vi "Update_Ch_data_file.vi"(5 "Range":enum16{"All Ch data", "The last few rows"}(ring), 7 "Channel to search on":string, 8 "Start of read offset (chars.: 0)":i32, 9 "New Row values":string[](array[string]), 10 "Present Channels":string[](array[string]), 11 "Filename":path) -> ()   [LabVIEW 2014]
panel:
  out "exists?":bool
  out "Merged?":bool
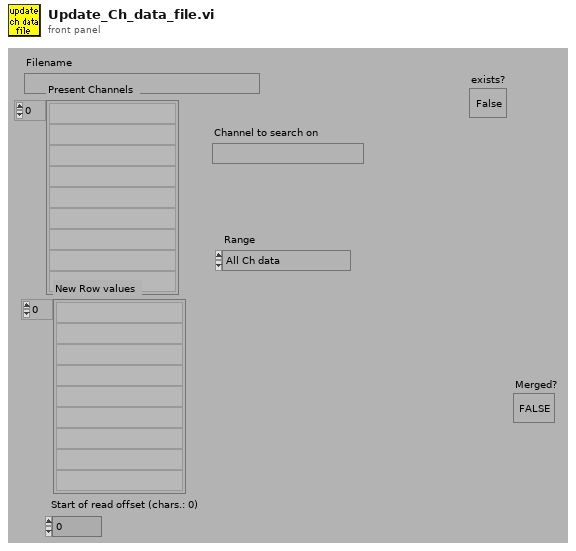
[diagram p1: front panel]
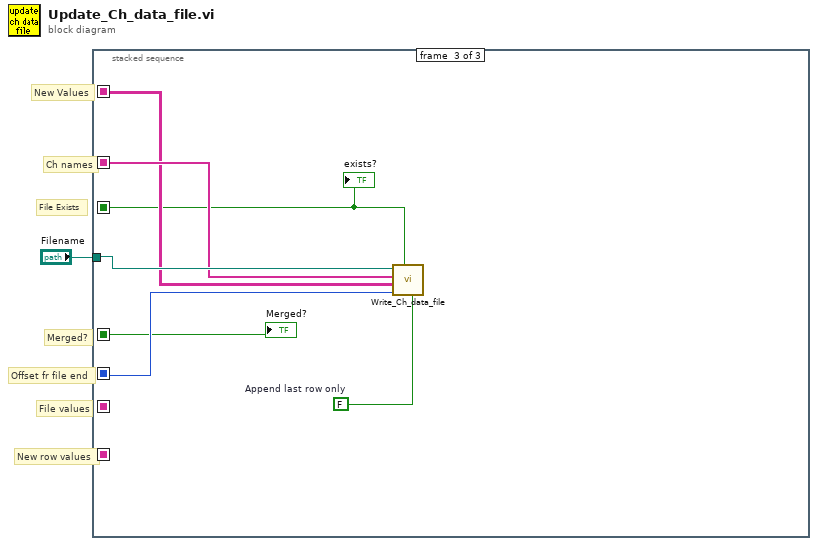
[diagram p0: block diagram]
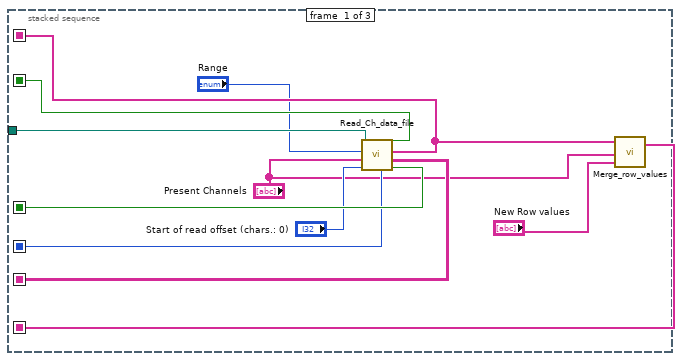
[diagram p2: hidden frame]
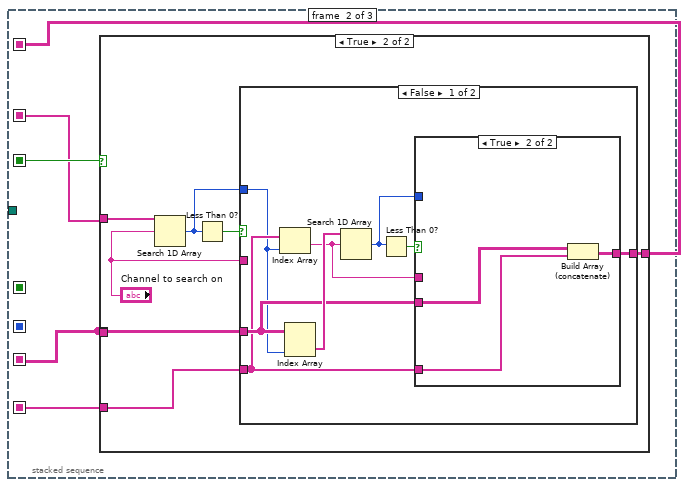
[diagram p3: hidden frame]
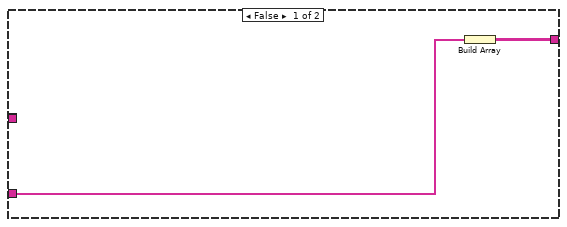
[diagram p4: hidden frame]
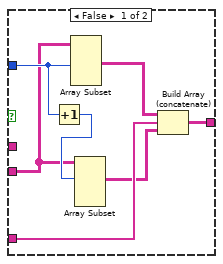
[diagram p5: hidden frame]
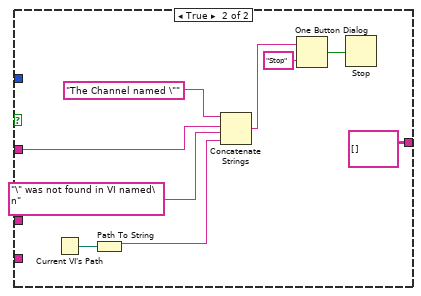
[diagram p6: hidden frame]
diagram:
  # "New row values"
  # "New Values"
  # "File values"
  # "Offset fr file end"
  # "Ch names"
  # "File Exists"
  # "Merged?"
  n1 = stacked-sequence {
    seq-local: [w8 _ _] -> [_ w13 _]
    seq-local: [_ w17 _] -> [_ _ w57]
    seq-local: [w12 _ _] -> [_ _ w54]
    seq-local: [w11 _ _] -> [_ w16 w56]
    seq-local: [w4 _ _] -> [_ w15 w59]
    seq-local: [w9 _ _] -> [_ _ w58]
    seq-local: [w3 _ _] -> [_ w14 _]
    tunnel: "Filename" -> [w10 _ w60]
    frame #0 {
      n2 = call "Read_Ch_data_file.vi"("Start of read offset (chars.: 0)"="Start of read offset (chars.: 0)", "Present Channels"="Present Channels", "Output"="Range", "Filename"=w10) -> ("Merged?"=w12:bool, "Channel Values"=w8:string[][], "Merged Channels"=w4:string[], "exists?"=w11:bool, "Offset from File End"=w9:i32)  [unwired: 1 in]
      n3 = call "Merge_row_values.vi"("Present Row values"="New Row values", "Present Channels"="Present Channels", "Desired Channels"=w4) -> ("Desired Row values"=w3:string[])  [unwired: 1 out]
    }
    frame #1 {
      n4 = case shown="True" w16 {
        tunnel: w15 -> [_ w24]
        tunnel: w13 -> [_ w23]
        tunnel: w14 -> [w18 w22]
        tunnel: [w19 w21] -> w17
        tunnel: w13 -> [_ _]
        frame False {
          n5 = Build Array(w18) -> (w19:string[][])
        }
        frame True {
          n6 = Search 1D Array(1D array=w24, element="Channel to search on") -> (index of element=w25:i32)  [unwired: 1 out]
          n7 = Less Than 0?(x=w25) -> (x < 0?=w26:bool)
          n8 = case shown="False" w26 {
            tunnel: "Channel to search on" -> [_ w46]
            tunnel: w25 -> [w28 _]
            tunnel: w23 -> [w31 _]
            tunnel: w22 -> [w29 _]
            tunnel: [w30 string[][] []] -> w21
            frame False {
              n9 = Index Array(array=w29, index=w28) -> (element=w27:string)
              n10 = Index Array(array=w31, index (col)=w28) -> (element=w34:string[])  [unwired: 1 in]
              n11 = Search 1D Array(1D array=w34, element=w27) -> (index of element=w32:i32)  [unwired: 1 out]
              n12 = Less Than 0?(x=w32) -> (x < 0?=w33:bool)
              n13 = case shown="True" w33 {
                tunnel: w27 -> [_ _]
                tunnel: w32 -> [w39 _]
                tunnel: w31 -> [w37 w43]
                tunnel: w29 -> [w40 w42]
                tunnel: [w35 w44] -> w30
                frame False {
                  n14 = Increment(x=w39) -> (x+1=w38:i32)
                  n15 = Array Subset(array=w37, length (row)=w39) -> (w41:string[][])  [unwired: 3 in]
                  n16 = Array Subset(array=w37, index (row)=w38) -> (w36:string[][])  [unwired: 3 in]
                  n17 = Build Array (concatenate)(w41, w40, w36) -> (w35:string[][])
                }
                frame True {
                  n18 = Build Array (concatenate)(w43, w42) -> (w44:string[][])
                }
              }
            }
            frame True {
              n19 = Current VI's Path() -> (path=w51:path)
              n20 = Path To String(path=w51) -> (string=w50:string)
              n21 = Concatenate Strings("The Channel named \"" ("message"), w46, "\" was not found in VI named\n" ("Channel to search on"), w50) -> (w49:string)
              n22 = One Button Dialog(message=w49, button name ("OK")="Stop") -> (true=w47:bool)
              n23 = Stop(stop? (T)=w47) -> ()
            }
          }
        }
      }
    }
    frame #2 {
      w55 = FALSE  # Append last row only
      n24 = call "Write_Ch_data_file.vi"("Append last row only"=w55, "exists?"=w56, "Write offset fr file end"=w58, "Channel Values"=w57, "Channel names"=w59, "Filename"=w60) -> ()  [unwired: 2 in, 4 out]
      "exists?" <- w56
      "Merged?" <- w54
    }
  }
